vi "GetText.vi"(8 "error in":errorcluster, 11 "node in":refnum<class "Initialization.lvclass">) -> (0 "error out":errorcluster, 1 "additional text":string, 2 "text":string, 3 "node out":refnum<class "Initialization.lvclass">, 4 "glyph":string)   [LabVIEW 2019, in "Initialization.lvclass"]
doc: "Returns the text representation of the node used for the tree control."
uses:
  Initialization.lvclass
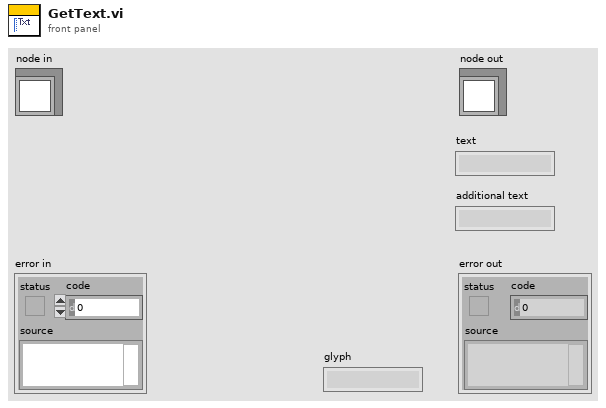
[diagram p1: front panel]
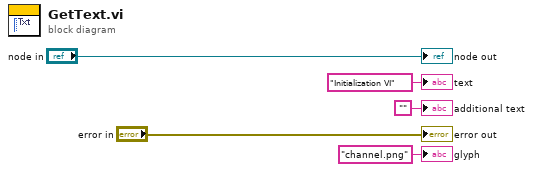
[diagram p0: block diagram]
diagram:
  "error out" <- "error in"
  "node out" <- "node in"
  "text" <- "Initialization VI" ("text")
  "additional text" <- ""
  "glyph" <- "channel.png" ("glyph")
